vi "ZDS1104 Read FREQ.vi"(8 "error in":errorcluster caption="错误输入", 11 "MyIndex":u8) -> (0 "error out":errorcluster caption="错误输出", 2 "FREQ_result":dbl)   [LabVIEW 2015]
uses:
  ZhiYuan ZDS Series for TCP/ZhiYuan ZDS Series for TCP.lvlib
panel:
  out "VISA":refnum<visa-resource-name> caption="VISA资源名称输出"
  out "读取缓冲区":string
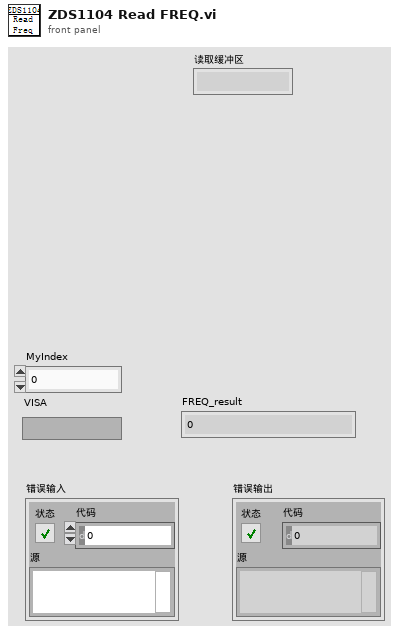
[diagram p1: front panel]
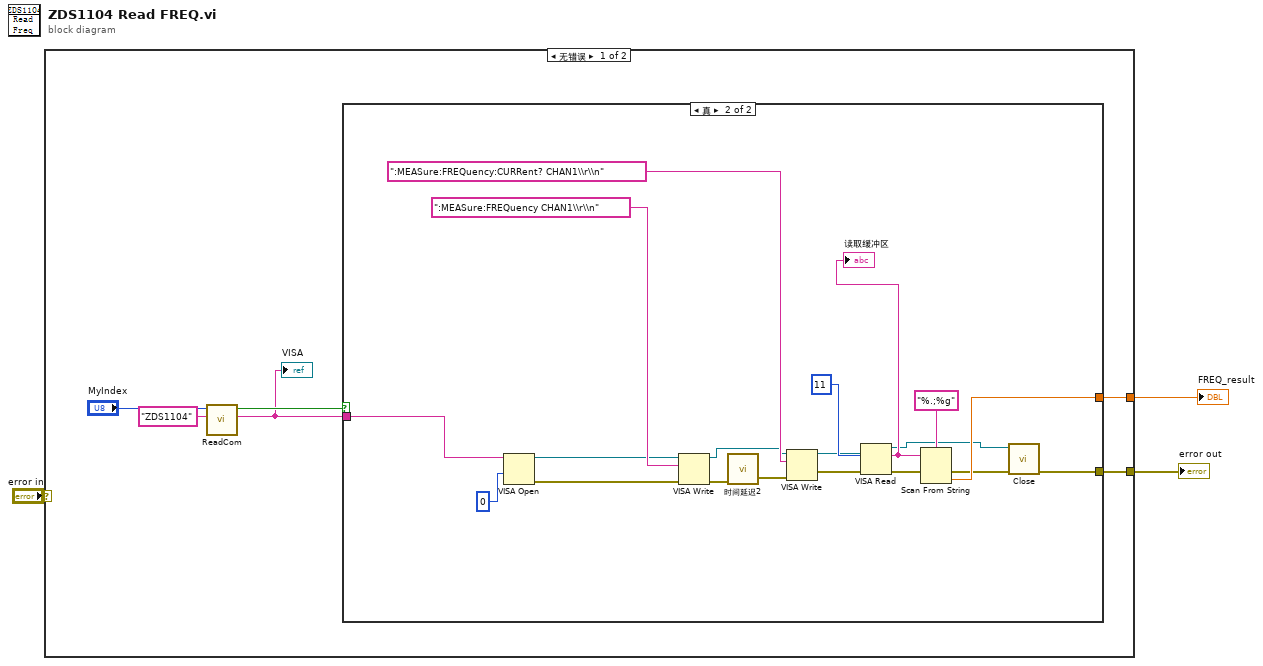
[diagram p0: block diagram]
diagram:
  n1 = case shown="无错误" "error in" {
    tunnel: [w9 _] -> w3
    tunnel: [w8 _] -> w2
    frame No Error {
      n2 = call "ReadCom.vi"("仪器名称"="ZDS1104", "MyIndex"="MyIndex") -> ("COM"=w4:string, "OK?"=w5:bool)  [unwired: 7 in, 1 out]
      "VISA" <- w4
      n3 = case shown="真" w5 {
        tunnel: [_ w28] -> w9
        tunnel: [_ w11] -> w8
        tunnel: w4 -> [_ w15]
        frame False {
        }
        frame True {
          n4 = VISA Open(access mode=u32 0, VISA resource name=w15) -> (VISA resource name=w14:refnum<visa-resource-name>, error out=w13:errorcluster)  [unwired: 3 in]
          n5 = VISA Write(VISA resource name=w14, write buffer=":MEASure:FREQuency CHAN1\\r\\n", error in (no error)=w13) -> (VISA resource name out=w17:refnum<visa-resource-name>, error out=w19:errorcluster)  [unwired: 1 out]
          n6 = call "时间延迟2"("error in (no error)"=w19) -> ("error out"=w18:errorcluster)  [unwired: 10 in]
          n7 = VISA Write(VISA resource name=w17, write buffer=":MEASure:FREQuency:CURRent? CHAN1\\r\\n", error in (no error)=w18) -> (VISA resource name out=w25:refnum<visa-resource-name>, error out=w24:errorcluster)  [unwired: 1 out]
          n8 = VISA Read(VISA resource name=w25, byte count=u32 11, error in (no error)=w24) -> (VISA resource name out=w10:refnum<visa-resource-name>, read buffer=w22:string, error out=w27:errorcluster)  [unwired: 1 out]
          "读取缓冲区" <- w22
          n9 = Scan From String(format string="%.;%g", input string=w22, error in=w27) -> (error out=w12:errorcluster, output 1=w28:dbl)  [unwired: 2 in, 2 out]
          n10 = call "Close.vi"("error in (no error)"=w12, "VISA resource name"=w10) -> ("error out"=w11:errorcluster)  [unwired: 9 in]
        }
      }
    }
    frame Error {
    }
  }
  "FREQ_result" <- w3
  "error out" <- w2
